vi "Configuration - Load INI File.vi"(8 "error in":errorcluster, 11 "configuration file path":path) -> (0 "error out":errorcluster, 3 "Carrier Configuration Out":T1)   [LabVIEW 2017, in "Communications Library.lvlib"]
doc: "Reads configuration data from an INI file, and stores that information in a functional global variable."
uses:
  Communications Library.lvlib
  Typedefs/DTACQ Module Carrier Configuration--Cluster.ctl
  Typedefs/DTACQ Module Configuration--Cluster.ctl
  Typedefs/DTACQ Device Type--Enum.ctl
  Typedefs/Functional Global Variable Action--Enum.ctl
  <vilib>/Utility/config.llb/Read Key (String).vi
  <vilib>/Utility/config.llb/NI_LVConfig.lvlib
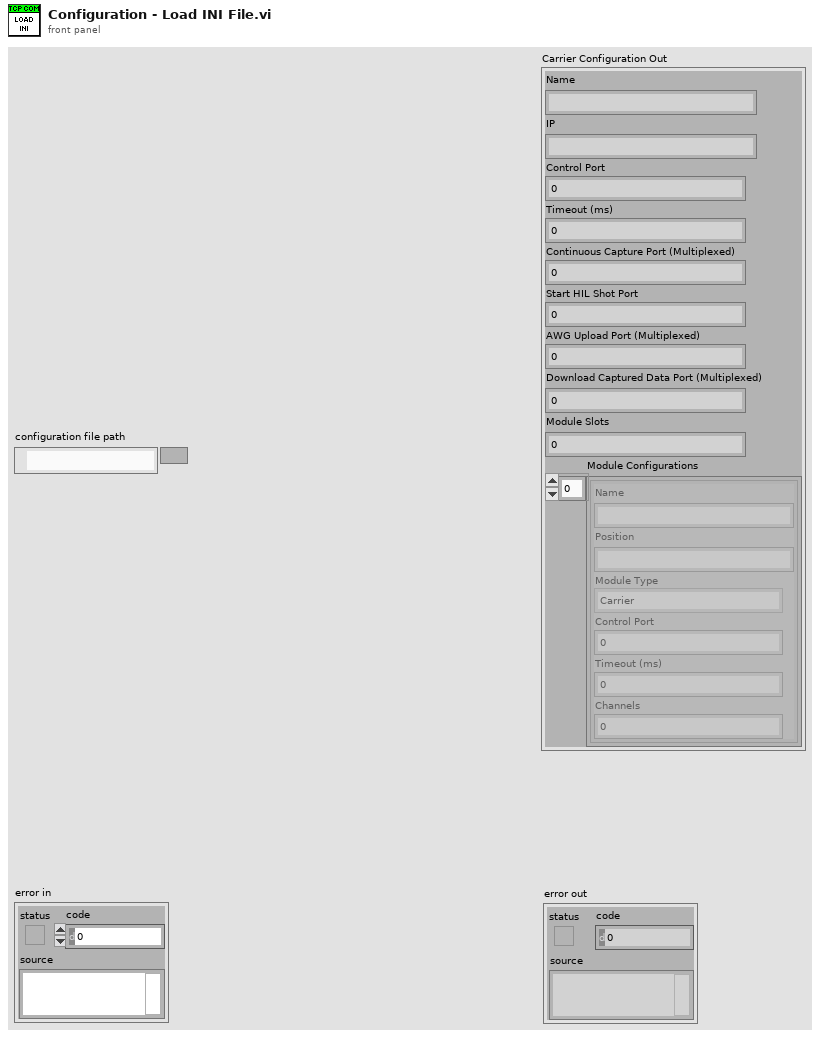
[diagram p1: front panel]
types:
  T1 = typedef "Communications Library.lvlib/DTACQ Module Carrier Configuration--Cluster.ctl" = cluster{"Name":string, "IP":string, "Control Port":i32, "Timeout (ms)":i32, "Continuous Capture Port (Multiplexed)":i32, "Start HIL Shot Port":i32, "AWG Upload Port (Multiplexed)":i32, "Download Captured Data Port (Multiplexed)":i32, "Module Slots":i32, "Module Configurations":T2[]}
  T2 = typedef "Communications Library.lvlib/DTACQ Module Configuration--Cluster.ctl" = cluster{"Name":string, "Position":string, "Module Type":T3, "Control Port":i32, "Timeout (ms)":i32, "Channels":i32}
  T3 = typedef "Communications Library.lvlib/DTACQ Device Type--Enum.ctl" = enum16{"Carrier", "Analog In Module", "Analog Out Module", "Generic Module"}
  T4 = typedef "NI_LVConfig.lvlib/Config Data RefNum.ctl" = refnum<k1>
  T5 = typedef "Communications Library.lvlib/Functional Global Variable Action--Enum.ctl" = enum16{"Initialise", "Write Module Config", "Write Carrier Config", "Read"}
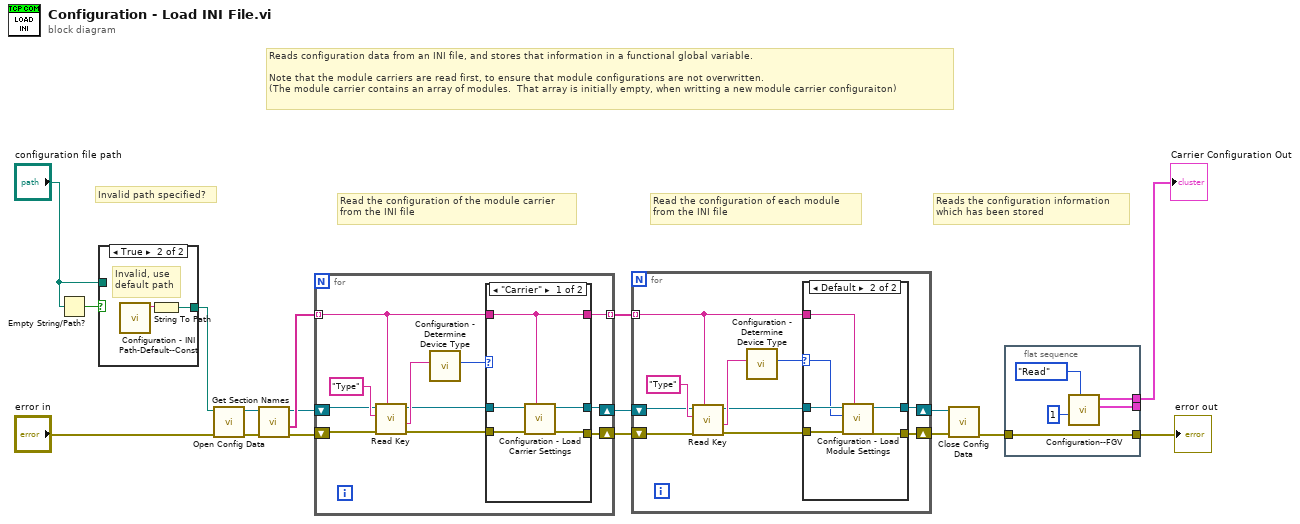
[diagram p0: block diagram]
diagram:
  # "Reads the configuration information\nwhich has been stored"
  # "Reads configuration data from an INI file, and stores that information in a functional global variable.\n\nNote that the module carriers are read first, to ensure that module configurations are not overwritten.\n(The module carrier contains an array of modules.  That array is initially empty, when writting a new module carrier configuraiton)"
  # "Read the configuration of each module\nfrom the INI file"
  # "Read the configuration of the module carrier\nfrom the INI file"
  # "Invalid path specified?"
  n1 = Empty String/Path?(string/path="configuration file path") -> (empty?=w3:bool)
  n2 = case shown="True" w3 {
    tunnel: [w18 w19] -> w1
    tunnel: "configuration file path" -> [w18 _]
    frame False {
      # "Valid path"
    }
    frame True {
      # "Invalid, use\ndefault path"
      n3 = call "Configuration - INI Path-Default--Const.vi"() -> ("Default INI Path"=w20:string)  [unwired: 11 in]
      n4 = String To Path(string=w20) -> (path=w19:path)
    }
  }
  n5 = call <vilib>:"Open Config Data.vi"("error in (no error)"="error in", "configuration file path"=w1) -> ("error out"=w16:errorcluster, "refnum"=w17:T4)  [unwired: 7 in, 1 out]
  n6 = call <vilib>:"Get Section Names.vi"("error in (no error)"=w16, "refnum"=w17) -> ("error out"=w13:errorcluster, "section names"=w15:string[], "refnum out"=w14:T4)  [unwired: 7 in]
  n7 = for {
    shift-right: [w24] -> w11
    shift-left: w14 -> [w29]
    shift-right: [w23] -> w12
    shift-left: w13 -> [w28]
    tunnel: w15 -> [w21] mode=indexing
    tunnel: [w22] -> w10 mode=indexing
    n8 = call-poly <vilib>:"Read Key.vi"("section"=w21, "error in (no error)"=w28, "key"="Type", "refnum"=w29) -> ("error out"=w26:errorcluster, "value"=w31:string, "refnum out"=w27:T4)  [unwired: 4 in, 1 out]
    n9 = call "Configuration - Determine Device Type.vi"("Type String In"=w31) -> ("Device Type Out"=w25:T3)  [unwired: 10 in]
    n10 = case shown="\"Carrier\"" w25 {
      tunnel: w27 -> [w36 w39]
      tunnel: w26 -> [w35 w38]
      tunnel: [w33 w39] -> w24
      tunnel: [w34 w38] -> w23
      tunnel: w21 -> [w32 w37]
      tunnel: [w32 w37] -> w22
      frame "Carrier" {
        n11 = call "Configuration - Load Carrier Settings.vi"("Section"=w32, "error in"=w35, "Refnum in"=w36) -> ("error out"=w34:errorcluster, "refnum out"=w33:T4)  [unwired: 7 in]
      }
      frame Default {
      }
    }
  }
  n12 = for {
    shift-right: [w42] -> w9
    shift-left: w11 -> [w47]
    shift-right: [w41] -> w7
    shift-left: w12 -> [w46]
    tunnel: w10 -> [w40] mode=indexing
    n13 = call-poly <vilib>:"Read Key.vi"("section"=w40, "error in (no error)"=w46, "key"="Type", "refnum"=w47) -> ("error out"=w44:errorcluster, "value"=w49:string, "refnum out"=w45:T4)  [unwired: 4 in, 1 out]
    n14 = call "Configuration - Determine Device Type.vi"("Type String In"=w49) -> ("Device Type Out"=w43:T3)  [unwired: 10 in]
    n15 = case shown="Default" w43 {
      selector: w43 -> [_ w52]
      tunnel: w45 -> [w51 w56]
      tunnel: w44 -> [w50 w57]
      tunnel: [w51 w55] -> w42
      tunnel: [w50 w54] -> w41
      tunnel: w40 -> [_ w53]
      frame "Carrier" {
      }
      frame Default {
        n16 = call "Configuration - Load Module Settings.vi"("section"=w53, "error in"=w57, "Device Type"=w52, "Refnum in"=w56) -> ("error out"=w54:errorcluster, "Refnum out"=w55:T4)  [unwired: 6 in]
      }
    }
  }
  n17 = call <vilib>:"Close Config Data.vi"("error in (no error)"=w7, "refnum"=w9) -> ("error out"=w5:errorcluster)  [unwired: 8 in, 1 out]
  n18 = flat-sequence {
    tunnel: [w61] -> w6
    tunnel: [w60] -> _
    tunnel: w5 -> [w58]
    tunnel: [w58] -> w4
    frame #0 {
      n19 = call "Configuration--FGV.vi"("Functional Global Action"=Functional_Global_Variable_Action--Enum."Read", "Module Number"=1) -> ("Module Configuration Out"=w60:T2, "Carrier Configuration Out"=w61:T1)  [unwired: 8 in]
    }
  }
  "error out" <- w4
  "Carrier Configuration Out" <- w6
